vi "System Error Cluster Replacement.vi"(8 "error in (no error)":errorcluster) -> (0 "error out":errorcluster)   [LabVIEW 2017]
doc: "Tool Menu Plugin - Run System Error Cluster Replacement."
types:
  T1 = enum32{"Invalid", "Standard", "Closed", "Hidden", "Minimized", "Maximized"}
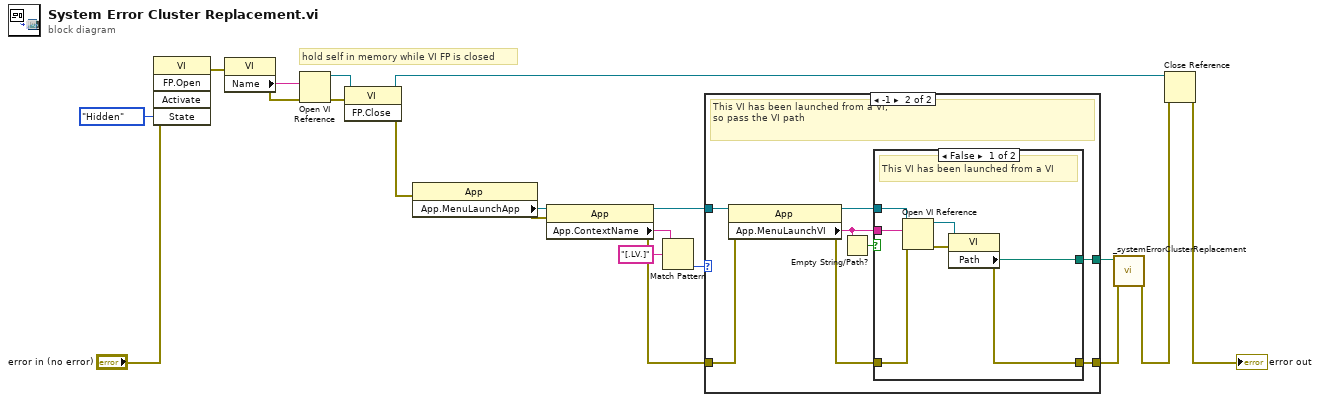
[diagram p0: block diagram]
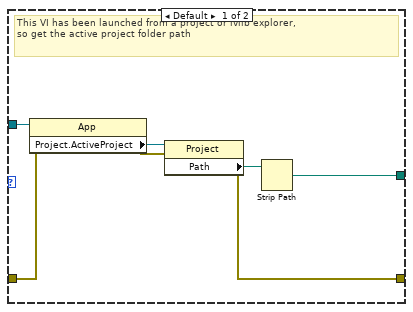
[diagram p2: hidden frame]
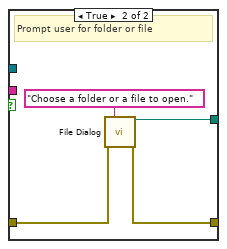
[diagram p3: hidden frame]
diagram:
  # "hold self in memory while VI FP is closed"
  n1 = invoke class="VI" method="FP.Open"(error in="error in (no error)", "State"=T1."Hidden") -> (error out=w2:errorcluster)  [unwired: 3 in, 4 out]
  n2 = property class="VI"(error in=w2) -> (error out=w9:errorcluster, "Name"=w13:string)  [unwired: 1 in, 1 out]
  n3 = Open VI Reference(vi path=w13, error in (no error)=w9) -> (vi reference=w12:refnum<vi>, error out=w11:errorcluster)  [unwired: 4 in]
  n4 = invoke class="VI" method="FP.Close"(reference=w12, error in=w11) -> (reference out=w3:refnum<vi>, error out=w1:errorcluster)  [unwired: 1 in, 1 out]
  n5 = property class="App"(error in=w1) -> (error out=w17:errorcluster, "App.MenuLaunchApp"=w20:refnum<vi>)  [unwired: 1 in, 1 out]
  n6 = property class="App"(reference=w20, error in=w17) -> (reference out=w15:refnum<vi>, error out=w14:errorcluster, "App.ContextName"=w19:string)
  n7 = Match Pattern(string=w19, regular expression="[.LV.]") -> (offset past match=w16:i32)  [unwired: 1 in, 3 out]
  n8 = case shown="-1" w16 {
    tunnel: w15 -> [w25 w35]
    tunnel: w14 -> [w24 w32]
    tunnel: [w23 w28] -> w4
    tunnel: [w21 w29] -> w6
    frame Default {
      # "This VI has been launched from a project or lvlib explorer, \nso get the active project folder path"
      n9 = property class="App"(reference=w25, error in=w24) -> (error out=w26:errorcluster, "Project.ActiveProject"=w27:refnum<vi>)  [unwired: 1 out]
      n10 = property class="Project"(reference=w27, error in=w26) -> (error out=w23:errorcluster, "Path"=w22:path)  [unwired: 1 out]
      n11 = Strip Path(path=w22) -> (stripped path=w21:path)  [unwired: 1 out]
    }
    frame -1 {
      # "This VI has been launched from a VI,\nso pass the VI path"
      n12 = property class="App"(reference=w35, error in=w32) -> (reference out=w30:refnum<vi>, error out=w31:errorcluster, "App.MenuLaunchVI"=w33:string)
      n13 = Empty String/Path?(string/path=w33) -> (empty?=w34:bool)
      n14 = case shown="False" w34 {
        tunnel: w33 -> [w42 _]
        tunnel: w31 -> [w40 w44]
        tunnel: [w37 w43] -> w28
        tunnel: w30 -> [w41 _]
        tunnel: [w36 w46] -> w29
        frame False {
          # "This VI has been launched from a VI"
          n15 = Open VI Reference(application reference (local)=w41, vi path=w42, error in (no error)=w40) -> (vi reference=w38:refnum<vi>, error out=w39:errorcluster)  [unwired: 3 in]
          n16 = property class="VI"(reference=w38, error in=w39) -> (error out=w37:errorcluster, "Path"=w36:path)  [unwired: 1 out]
        }
        frame True {
          # "Prompt user for folder or file"
          n17 = call "File Dialog"("prompt"="Choose a folder or a file to open.", "error in"=w44) -> ("selected path"=w46:path, "error out"=w43:errorcluster)  [unwired: 10 in, 2 out]
        }
      }
    }
  }
  n18 = call "_systemErrorClusterReplacement.vi"("error in (no error)"=w4, "Folder Path"=w6) -> ("error out"=w5:errorcluster)  [unwired: 9 in]
  n19 = Close Reference(reference=w3, error in (no error)=w5) -> (error out=→"error out":errorcluster)
